vi "Update Price.vi"(8 "error in (no error)":errorcluster, 10 "Price":dbl format="%#_13g", 11 "Name":string) -> (0 "error out":errorcluster)   [LabVIEW 2020, in "SQLITE Inventory.lvlib"]
doc: "Updates the price value of a single product according to the given name."
uses:
  SQLITE Inventory.lvlib
  <vilib>/drjdpowell/SQLite Library/SQL Connection/Open (path).vi
  <vilib>/drjdpowell/SQLite Library/SQL Connection/Open (string).vi
  <vilib>/AdvancedString/Path To Command Line String.vi
  <vilib>/drjdpowell/SQLite Library/SQL Connection/Execute SQL (No results).vi
  <vilib>/drjdpowell/SQLite Library/SQL Connection/Connection.lvclass
  <vilib>/drjdpowell/SQLite Library/SQLite.lvlib
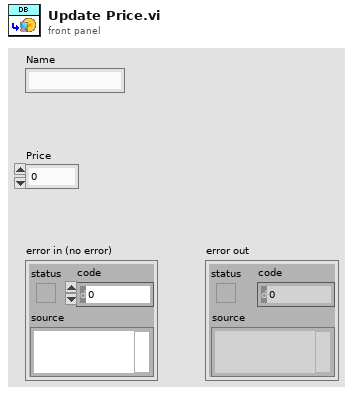
[diagram p1: front panel]
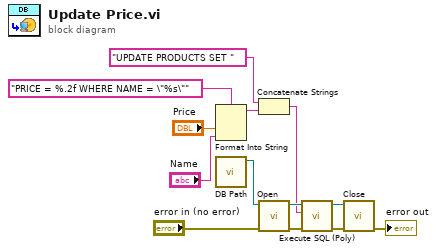
[diagram p0: block diagram]
diagram:
  n1 = Format Into String(format string="PRICE = %.2f WHERE NAME = \"%s\"", "Price", "Name") -> (resulting string=w6:string)  [unwired: 2 in, 1 out]
  n2 = call "DB Path.vi"() -> ("DB Path"=w9:path)  [unwired: 11 in]
  n3 = Concatenate Strings("UPDATE PRODUCTS SET " ("SQL"), w6) -> (w5:string)
  n4 = call-poly <vilib>:"Open.vi"("error in (no error)"="error in (no error)", "db file"=w9) -> ("error out"=w11:errorcluster, "SQLite Connection"=w13:refnum<class "Connection.lvclass">)  [unwired: 8 in]
  n5 = call-poly <vilib>:"Execute SQL (Poly).vi"("error in (no error)"=w11, "SQL"=w5, "SQLite Connection in"=w13) -> ("error out"=w10:errorcluster, "SQLite Connection"=w12:refnum<class "Connection.lvclass">)  [unwired: 7 in]
  n6 = call-dynamic "Close.vi"("error in (no error)"=w10, "SQLite Connection in"=w12) -> ("error out"=→"error out":errorcluster)  [unwired: 9 in]
